vi "welcome.vi"(2 "error in (no error)":errorcluster) -> (0 "error out":errorcluster, 1 "Slide":u8(slide) scale=0.0..100.0)   [LabVIEW 2014]
panel:
  # "MENSAJE DE BIENVENIDA"
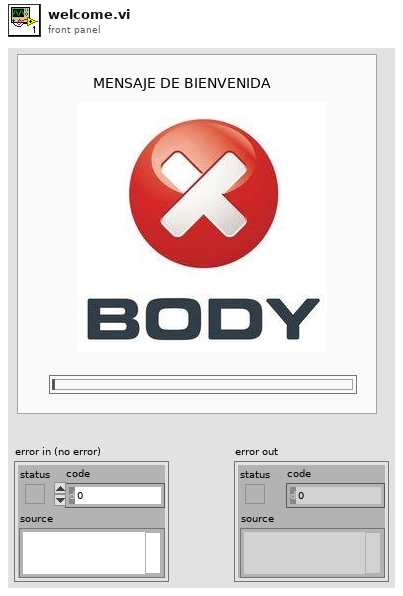
[diagram p1: front panel]
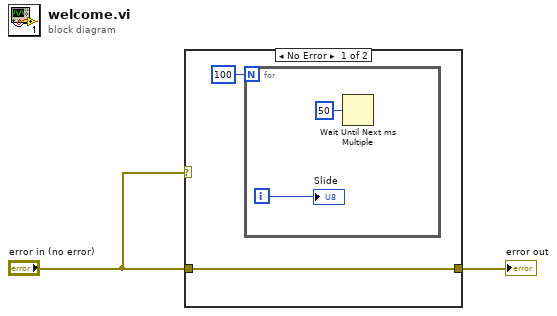
[diagram p0: block diagram]
diagram:
  n1 = case shown="No Error" "error in (no error)" {
    tunnel: "error in (no error)" -> [w3 w7]
    tunnel: [w3 w7] -> w1
    frame No Error {
      n2 = for {
        N: 100 -> [_]
        i -> [w5]
        n3 = Wait Until Next ms Multiple(millisecond multiple=u32 50) -> ()  [unwired: 1 out]
        "Slide" <- w5
      }
    }
    frame Error {
    }
  }
  "error out" <- w1
